vi "AvoidFunc.vi"() -> ()   [LabVIEW 2016, in "Team234_Project5.lvrbt"]
uses:
  Team234_Project5.lvrbt
  <vilib>/NXT/Block Support/NXT_InputPort.ctl
  <vilib>/NXT/Subs/LVHSConnector.ctl
  <vilib>/NXT/LegoClasses/BrickReference/BrickReference.lvclass
  <vilib>/NXT/Block Support/NXT_OutputPort.ctl
  <vilib>/NXT/Dual Mode Library/Sensors/EV3_Ultrasonic_IN.vi
  <vilib>/NXT/NXTIO Xnodes/NXTIONodeSubVIs/NXTStopMotors.vi
  <vilib>/NXT/NXTIO Xnodes/NXTIONodeSubVIs/NXTMoveMotors.vi
  <vilib>/NXT/Dual Mode Library/Waits/Wait_Num.vi
  <vilib>/NXT/NXTIO Xnodes/AddressXNode/NXTIOAddress.xnode
  <vilib>/NXT/NXTIO Xnodes/NXTIOXNode/NXTIO.xnode
panel:
  in  "Time (1 sec) 9":sgl=1.0
  in  "Time (1 sec) 8":sgl=1.0
  in  "Time (1 sec) 7":sgl=1.0
  in  "Time (1 sec) 6":sgl=1.0
  in  "Time (1 sec) 5":sgl=1.0
  in  "Time (1 sec) 4":sgl=1.0
  in  "Time (1 sec) 3":sgl=1.0
  in  "Time (1 sec) 2":sgl=1.0
  in  "Time (1 sec)":sgl=1.0
  in  "Power POSITIVE":i8=75
  in  "Power NEGATIVE":i8=75
  out "Inches (Output)":sgl
  in  "NXT/EV3":T1
  in  "Sensor Port (3)":T2 items=["Port 1", "Port 2", "Port 3", "Port 4"]
  # "Turn 1 Timer M2"
  # "Turn 1 Timer M1"
  # "Forward Timers"
  # "Turn 3 Timer M2"
  # "Turn 2 Timer M2"
  # "Turn 3 Timer M1"
  # "Turn 2 Timer M1"
  # "Turn FInal M1"
  # "Turn Final M2"
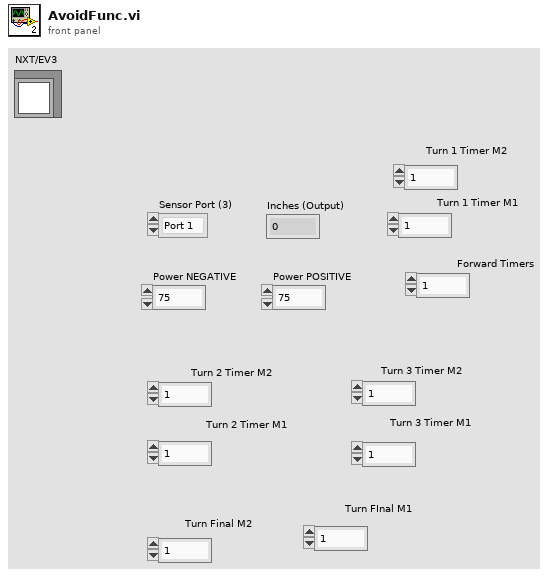
[diagram p1: front panel]
types:
  T1 = typedef "LVHSConnector.ctl" = refnum<class "BrickReference.lvclass">
  T2 = typedef "NXT_InputPort.ctl" = u32
  T3 = typedef "NXT_OutputPort.ctl" = u8
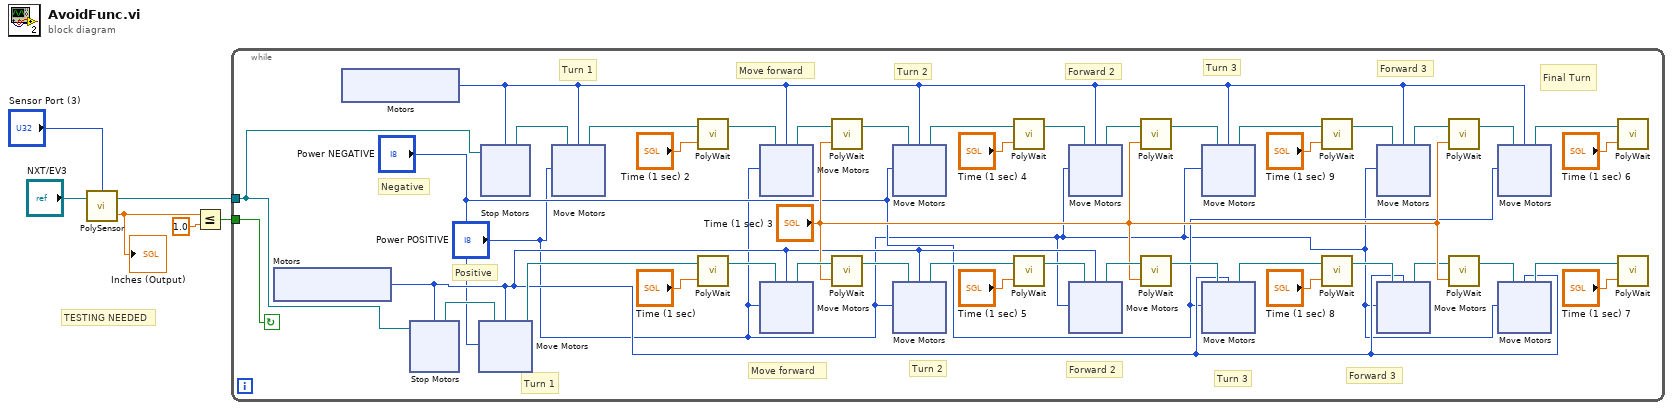
[diagram p0: block diagram]
diagram:
  # "TESTING NEEDED"
  n1 = call-poly <vilib>:"PolySensor.vi"("NXT/EV3"="NXT/EV3", "Port (Port 1)"="Sensor Port (3)") -> ("Inches"=w3:sgl, "NXT/EV3"=w1:T1)  [unwired: 1 in]
  "Inches (Output)" <- w3
  n2 = Less Or Equal?(x=w3, y=sgl 1.0) -> (x <= y?=w4:bool)
  n3 = while {
    tunnel: w4 -> [w49]
    tunnel: w1 -> [w48]
    stop <- w49 continue-if-true
    # "Final Turn"
    # "Forward 3"
    # "Forward 3"
    # "Turn 3"
    # "Turn 3"
    # "Forward 2"
    # "Forward 2"
    # "Turn 1"
    # "Turn 2"
    # "Turn 2"
    # "Move forward"
    # "Move forward"
    # "Turn 1"
    # "Negative"
    # "Positive"
    n4 = xnode "Motors"() -> ("Motor"=w13:T3)
    n5 = xnode "Motors"() -> ("Motor"=w14:T3)
    n6 = xnode "Stop Motors"("Motors"=w13, "NXT/EV3"=w48) -> ("NXT/EV3"=w46:T1)
    n7 = xnode "Move Motors"("Power/Speed 1"="Power NEGATIVE", "Motors"=w13, "NXT/EV3"=w46) -> ("NXT/EV3"=w44:T1)
    n8 = xnode "Stop Motors"("Motors"=w14, "NXT/EV3"=w48) -> ("NXT/EV3"=w47:T1)
    n9 = xnode "Move Motors"("Power/Speed 1"="Power POSITIVE", "Motors"=w14, "NXT/EV3"=w47) -> ("NXT/EV3"=w45:T1)
    n10 = call-poly <vilib>:"PolyWait.vi"("Time (1 sec)"="Time (1 sec) 2", "NXT/EV3"=w45) -> ("NXT/EV3"=w42:T1)  [unwired: 2 in]
    n11 = call-poly <vilib>:"PolyWait.vi"("Time (1 sec)"="Time (1 sec)", "NXT/EV3"=w44) -> ("NXT/EV3"=w43:T1)  [unwired: 2 in]
    n12 = xnode "Move Motors"("Power/Speed 1"="Power POSITIVE", "Motors"=w14, "NXT/EV3"=w42) -> ("NXT/EV3"=w41:T1)
    n13 = xnode "Move Motors"("Power/Speed 1"="Power POSITIVE", "Motors"=w13, "NXT/EV3"=w43) -> ("NXT/EV3"=w38:T1)
    n14 = call-poly <vilib>:"PolyWait.vi"("Time (1 sec)"="Time (1 sec) 3", "NXT/EV3"=w41) -> ("NXT/EV3"=w36:T1)  [unwired: 2 in]
    n15 = call-poly <vilib>:"PolyWait.vi"("Time (1 sec)"="Time (1 sec) 3", "NXT/EV3"=w38) -> ("NXT/EV3"=w37:T1)  [unwired: 2 in]
    n16 = xnode "Move Motors"("Power/Speed 1"="Power NEGATIVE", "Motors"=w14, "NXT/EV3"=w36) -> ("NXT/EV3"=w35:T1)
    n17 = xnode "Move Motors"("Power/Speed 1"="Power POSITIVE", "Motors"=w13, "NXT/EV3"=w37) -> ("NXT/EV3"=w31:T1)
    n18 = call-poly <vilib>:"PolyWait.vi"("Time (1 sec)"="Time (1 sec) 4", "NXT/EV3"=w35) -> ("NXT/EV3"=w34:T1)  [unwired: 2 in]
    n19 = call-poly <vilib>:"PolyWait.vi"("Time (1 sec)"="Time (1 sec) 5", "NXT/EV3"=w31) -> ("NXT/EV3"=w32:T1)  [unwired: 2 in]
    n20 = xnode "Move Motors"("Power/Speed 1"="Power POSITIVE", "Motors"=w14, "NXT/EV3"=w34) -> ("NXT/EV3"=w33:T1)
    n21 = xnode "Move Motors"("Power/Speed 1"="Power POSITIVE", "Motors"=w13, "NXT/EV3"=w32) -> ("NXT/EV3"=w26:T1)
    n22 = call-poly <vilib>:"PolyWait.vi"("Time (1 sec)"="Time (1 sec) 3", "NXT/EV3"=w33) -> ("NXT/EV3"=w28:T1)  [unwired: 2 in]
    n23 = call-poly <vilib>:"PolyWait.vi"("Time (1 sec)"="Time (1 sec) 3", "NXT/EV3"=w26) -> ("NXT/EV3"=w27:T1)  [unwired: 2 in]
    n24 = xnode "Move Motors"("Power/Speed 1"="Power POSITIVE", "Motors"=w14, "NXT/EV3"=w28) -> ("NXT/EV3"=w24:T1)
    n25 = xnode "Move Motors"("Power/Speed 1"="Power NEGATIVE", "Motors"=w13, "NXT/EV3"=w27) -> ("NXT/EV3"=w25:T1)
    n26 = call-poly <vilib>:"PolyWait.vi"("Time (1 sec)"="Time (1 sec) 9", "NXT/EV3"=w24) -> ("NXT/EV3"=w20:T1)  [unwired: 2 in]
    n27 = call-poly <vilib>:"PolyWait.vi"("Time (1 sec)"="Time (1 sec) 8", "NXT/EV3"=w25) -> ("NXT/EV3"=w21:T1)  [unwired: 2 in]
    n28 = xnode "Move Motors"("Power/Speed 1"="Power POSITIVE", "Motors"=w14, "NXT/EV3"=w20) -> ("NXT/EV3"=w19:T1)
    n29 = xnode "Move Motors"("Power/Speed 1"="Power POSITIVE", "Motors"=w13, "NXT/EV3"=w21) -> ("NXT/EV3"=w22:T1)
    n30 = call-poly <vilib>:"PolyWait.vi"("Time (1 sec)"="Time (1 sec) 3", "NXT/EV3"=w19) -> ("NXT/EV3"=w18:T1)  [unwired: 2 in]
    n31 = call-poly <vilib>:"PolyWait.vi"("Time (1 sec)"="Time (1 sec) 3", "NXT/EV3"=w22) -> ("NXT/EV3"=w17:T1)  [unwired: 2 in]
    n32 = xnode "Move Motors"("Power/Speed 1"="Power NEGATIVE", "Motors"=w14, "NXT/EV3"=w18) -> ("NXT/EV3"=w15:T1)
    n33 = xnode "Move Motors"("Power/Speed 1"="Power POSITIVE", "Motors"=w13, "NXT/EV3"=w17) -> ("NXT/EV3"=w16:T1)
    n34 = call-poly <vilib>:"PolyWait.vi"("Time (1 sec)"="Time (1 sec) 6", "NXT/EV3"=w15) -> ()  [unwired: 2 in, 1 out]
    n35 = call-poly <vilib>:"PolyWait.vi"("Time (1 sec)"="Time (1 sec) 7", "NXT/EV3"=w16) -> ()  [unwired: 2 in, 1 out]
  }
